vi "Insert2CouchDB.vi"(0 "value":dbl, 1 "title":string, 2 "name":string) -> ()   [LabVIEW 2011]
doc: "This example demonstrates how to use an event structure to post a message and pass data to the event structure using the PostLVUserEvent() function. The VI calls the dll using the Call Library Function Node, and the dll passes three messages to the event structure. A dialog window displays the data and remains open for 2 seconds. The dll is called in its own thread so it does not hang the UI thread."
uses:
  libs/AccCouchDB.dll
panel:
  out "write success":i32
  out "device registered":i32
  out "Ready":bool
  out "Size":dbl
  in  "Array":dbl[](array[numeric])
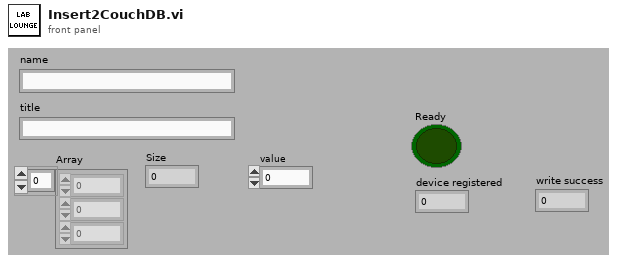
[diagram p1: front panel]
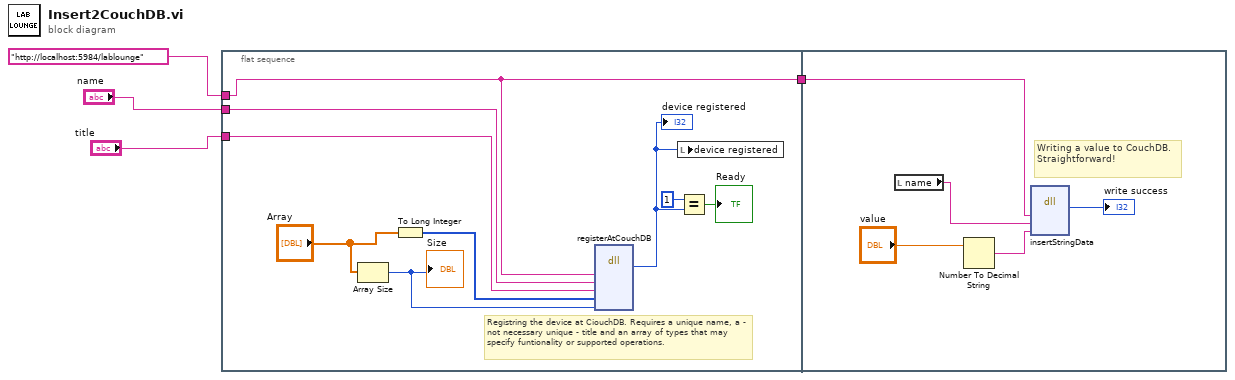
[diagram p0: block diagram]
diagram:
  n1 = flat-sequence {
    tunnel: "http://localhost:5984/lablounge" ("server") -> [w6]
    tunnel: [w6] -> w4
    tunnel: "name" -> [w11]
    tunnel: "title" -> [w10]
    tunnel: w4 -> [w14]
    frame #0 {
      # "Registring the device at CiouchDB. Requires a unique name, a - not necessary unique - title and an array of types that may specify funtionality or supported operations."
      n2 = Array Size(array="Array") -> (size(s)=w9:i32)
      "Size" <- w9
      n3 = To Long Integer(number="Array") -> (32bit integer=w7:i32[])
      n4 = dll-call lib="C:/projects/libs/AccCouchDB.dll" fn="registerAtCouchDB"("server"=w6, "name"=w11, "title"=w10, "types"=w7, "types_count"=w9) -> ("return type"=w5:i32)  [unwired: 8 in, 2 out]
      "device registered" <- w5
      n5 = local write "device registered"(w5) -> ()
      n6 = Equal?(x=1, y=w5) -> (x = y?=→"Ready":bool)
    }
    frame #1 {
      # "Writing a value to CouchDB. Straightforward!"
      n7 = local read "name"() -> (w16:string)
      n8 = Number To Decimal String(number="value") -> (decimal integer string=w15:string)  [unwired: 1 in]
      n9 = dll-call lib="C:/projects/libs/AccCouchDB.dll" fn="insertStringData"("server"=w14, "key"=w16, "value"=w15) -> ("return type"=→"write success":i32)  [unwired: 6 in, 2 out]
    }
  }
